vi "Read Vertical Scrollbar Visibility.vi"(9 "Pane in":refnum<class "Pane.lvclass">) -> (3 "Pane out":refnum<class "Pane.lvclass">, 4 "Vertical Scrollbar Visibility":T1(ring))   [LabVIEW 2014, in "Pane.lvclass"]
uses:
  Pane.lvclass
  Pane.lvclass/Pane.ctl
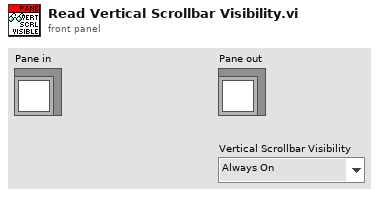
[diagram p1: front panel]
types:
  T1 = enum16{"Always On", "Always Off", "Off While Running"}
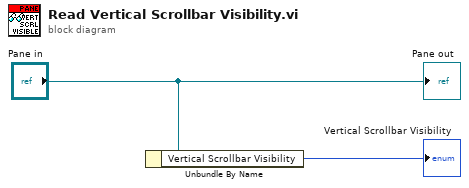
[diagram p0: block diagram]
diagram:
  n1 = Unbundle By Name("Pane in") -> ("Vertical Scrollbar Visibility"=→"Vertical Scrollbar Visibility":T1)
  "Pane out" <- "Pane in"
